vi "TREE_delete tree.vi"(8 "error in":errorcluster, 11 "Tree In":refnum<vi>) -> (0 "error out":errorcluster, 3 "Tree Out":refnum<vi>)   [LabVIEW 2011]
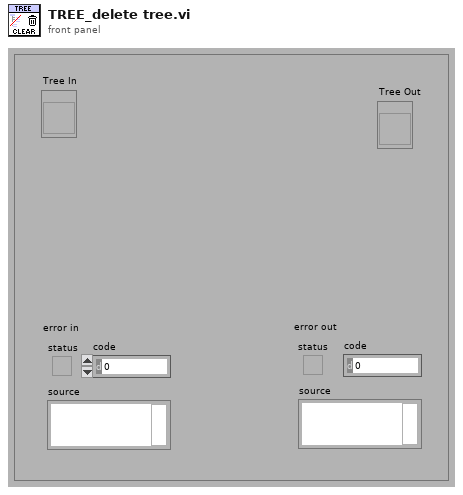
[diagram p1: front panel]
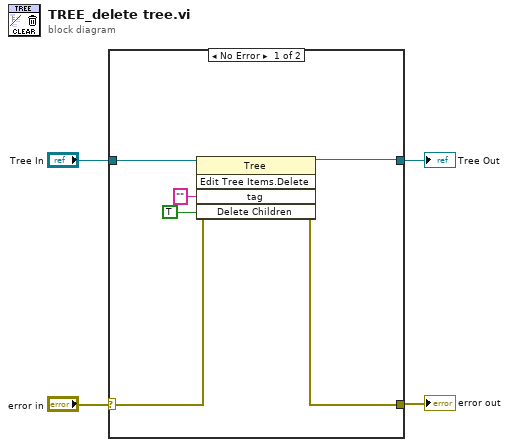
[diagram p0: block diagram]
diagram:
  n1 = case shown="No Error" "error in" {
    selector: "error in" -> [w7 w12]
    tunnel: "Tree In" -> [w8 w11]
    tunnel: [w5 w11] -> w3
    tunnel: [w6 w12] -> w2
    frame No Error {
      n2 = invoke class="Tree" method="Edit Tree Items.Delete"(reference=w8, error in=w7, "tag"="", "Delete Children"=TRUE) -> (reference out=w5:refnum<vi>, error out=w6:errorcluster)  [unwired: 1 in, 3 out]
    }
    frame Error {
      (unwired) string[] [] ("directory names")
      (unwired) path ""
      (unwired) "" ("name")
    }
  }
  "Tree Out" <- w3
  "error out" <- w2
